vi "main.vi"() -> ()   [LabVIEW 2009]
uses:
  subvi/activity_info.vi
  <vilib>/Utility/file.llb/Write To Spreadsheet File (DBL).vi
  <vilib>/Utility/sysdir.llb/System Directory Type.ctl
panel:
  in  "Do ANN analysis":bool
  in  "Analysis Upperbound (minutes)":dbl(slide)=1000.0 scale=0.0..30.0
  out "minutes left":dbl
  out "minutes of execution":dbl
  out "case 3":i32
  out "case 2":i32
  out "case 1":i32
  out "case 0":i32
  out "output 2":dbl[](array[slide]) scale=0.0..1.0
  out "Correlations":cluster{dbl[], "correlation array":dbl[]}(graph)
  in  "Slide":cluster{dbl, dbl}(slide)={0.0, 1.0} scale=0.0..1.0
  out "above threshold":dbl(slide) scale=0.0..1.0
  in  "Threshold":dbl(slide)=0.85 scale=0.0..1.0
  out "Analyzing":u8(slide) scale=0.0..100.0
  in  "analyze correlations":bool
  in  "Reference Signal":i32
  in  "Reference Signals":dbl[][](array[numeric])
  in  "Save Signal":bool
  in  "read weights":bool
  out "max amplitude":dbl(slide) scale=0.0..4.0
  in  "Path":path=path "E:/Sensor/data/Phase II Data/csv format/Ara/Ara Walking.csv"
  out "C":bool
  out "B":bool
  out "A":bool
  in  "write data":bool
  out "Fundamental frequency":dbl(slide) scale=0.0..6.0
  in  "Normalize":bool
  out "high":bool
  out "med":bool
  out "low":bool
  out "RMS":dbl(slide) scale=0.0..10.0
  in  "write to memory":bool
  out "activity output":u16(ring) items=["A", "B", "C", "D"]
  out "output":dbl[](array[slide]) scale=0.0..1.0
  in  "stop learning":bool
  out "Error (training)":dbl(graph)
  in  "Learning Rate":dbl(slide)=0.336734693877551 scale=0.0..1.0
  in  "Beta":dbl(slide)=1.0 scale=0.0..1.0
  in  "train":bool
  in  "Number of hidden neurons":i32(slide)=9 scale=0.0..20.0
  in  "delete state":bool
  in  "state":u32
  in  "activity":u16(ring) items=["A", "B", "C", "D", "E", "F", "G", "H"]
  in  "save state":bool
  in  "Tab Control":T1(tab)=enum."FFT on data 1"
  out "Time data on X',Y',Z'":T2(graph)
  out "FFT on X',Y',Z'":T3(graph)
  out "Filtered signal":dbl[](graph)
  out "Magnitude of time data":cluster{dbl[], dbl[]}(graph)
  out "activity states":T4(graph)
  in  "Sensor":u16(ring)=1 items=["Sensor 1", "Sensor 2", "Sensor 3"]
  in  "Sensor Type":u16(ring) items=["Acceleration", "Rotation"]
  in  "Sensor Brand":u16(ring)=1 items=["ADXL", "Kinetisense"]
  in  "End time (s) 1":dbl(slide)=10.0 scale=0.0..600.0
  in  "FFT interval (s) 1":dbl(slide)=4.0 scale=0.0..40.0
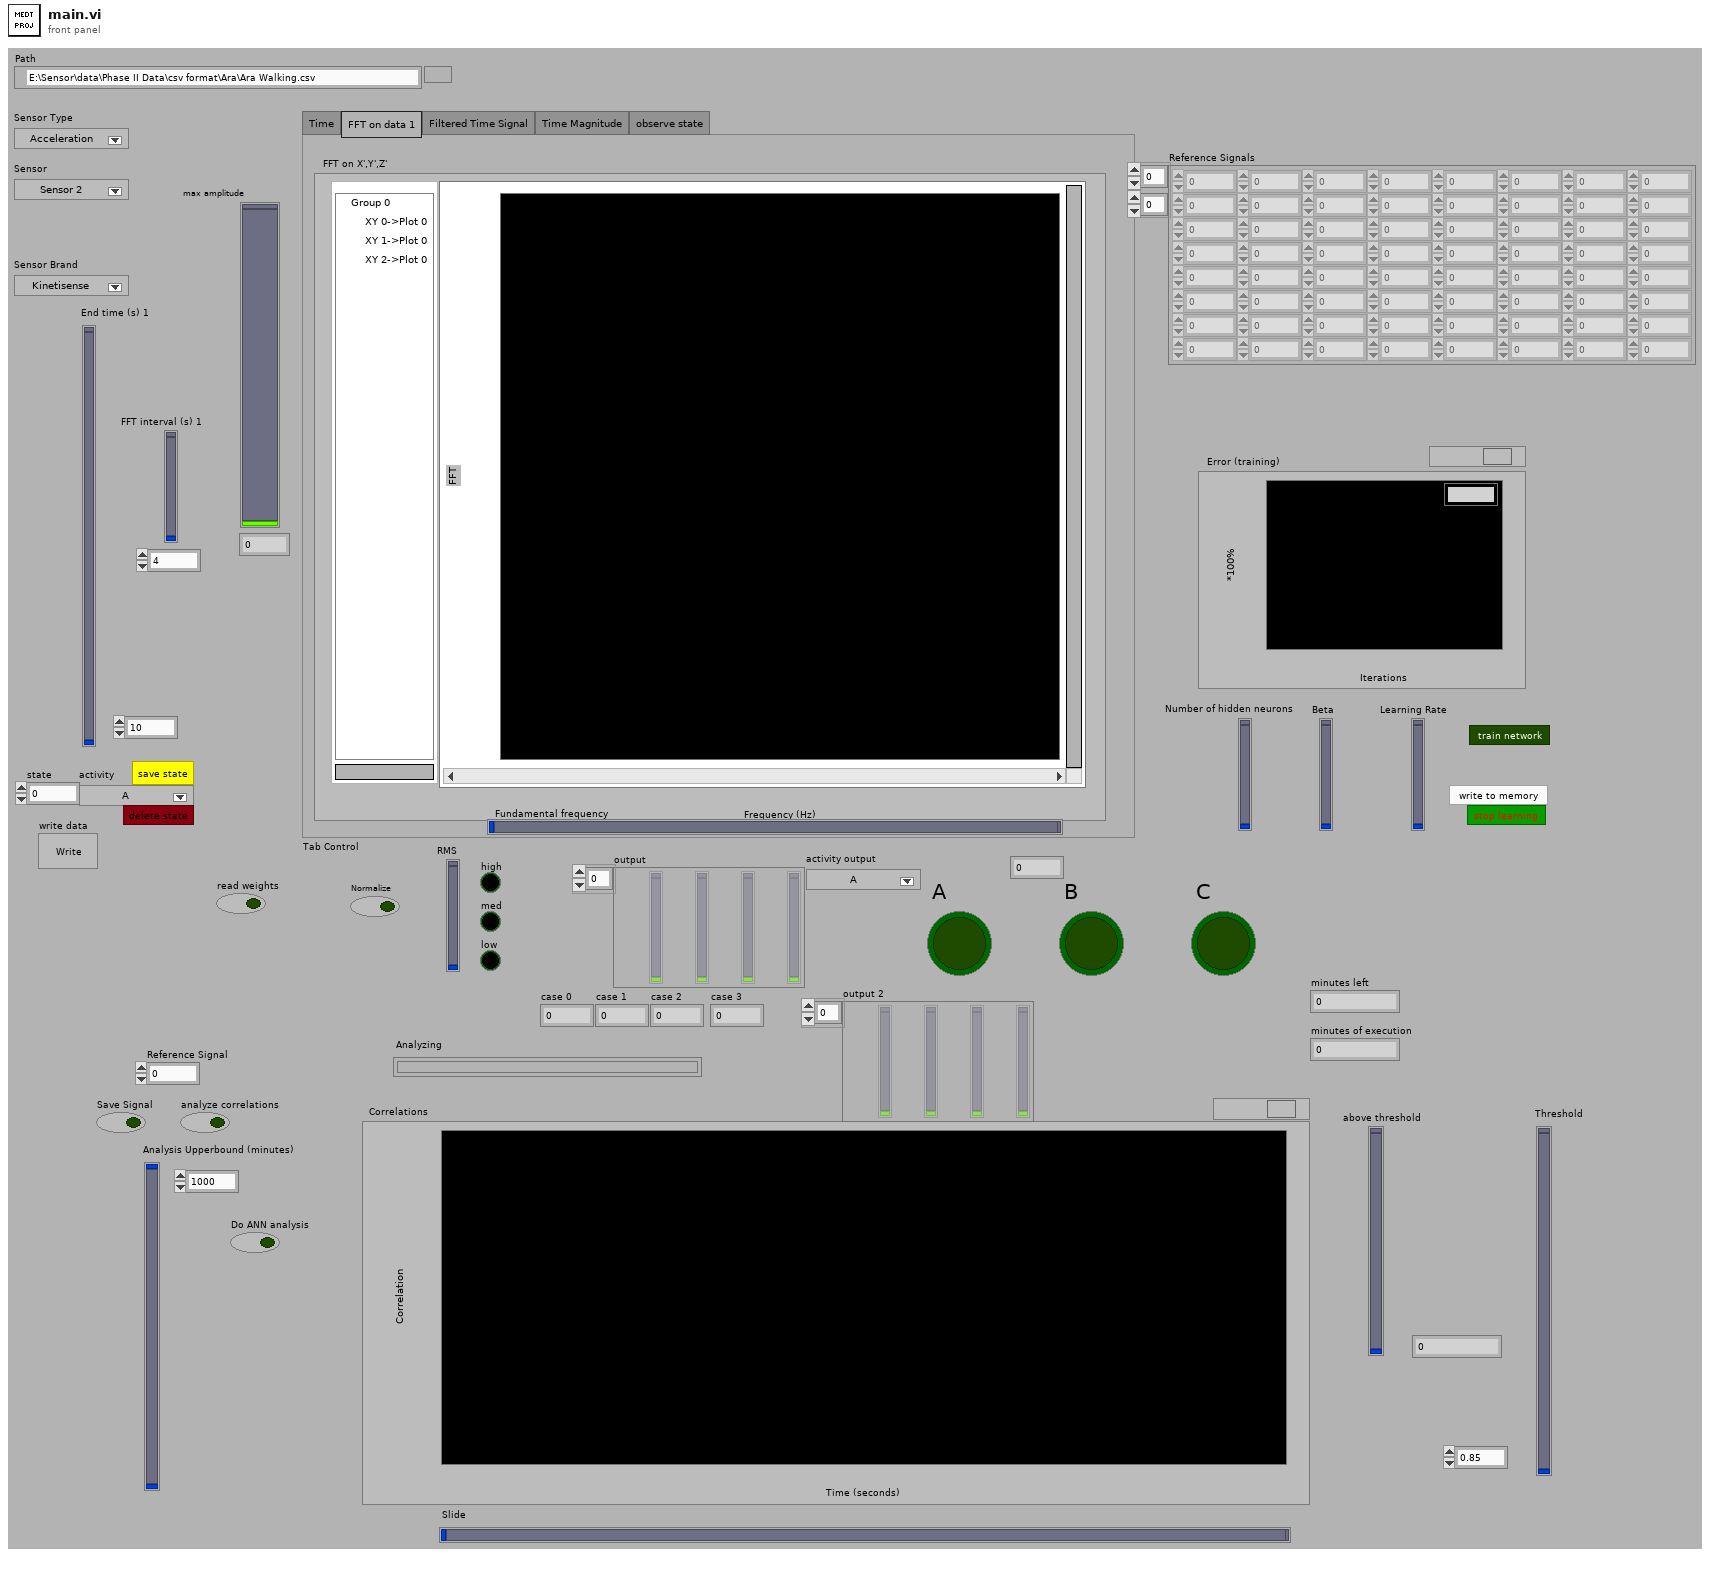
[diagram p1: front panel]
types:
  T1 = enum32{"Time", "FFT on data 1", "Filtered Time Signal", "Time Magnitude", "observe state"}
  T2 = cluster{cluster{dbl[], "Data out":dbl[]}, cluster{dbl[], "Data out":dbl[]}, cluster{dbl[], "Data out":dbl[]}}
  T3 = cluster{"XY Graph":cluster{dbl[], "magnitude":dbl[]}, "XY Graph":cluster{dbl[], "magnitude":dbl[]}, "XY Graph":cluster{dbl[], "magnitude":dbl[]}}
  T4 = cluster{cluster{dbl[], "Bicycling":dbl[]}, cluster{dbl[], "Bicycling":dbl[]}, cluster{dbl[], dbl[]}, cluster{dbl[], dbl[]}, cluster{dbl[], dbl[]}}
  T5 = typedef "System Directory Type.ctl" = i32
  T6 = cluster{"A":dbl[][], "B":dbl[][], "C":dbl[][], "D":dbl[][]}
  T7 = cluster{cluster{dbl[], dbl[]}, cluster{dbl[], dbl[]}, cluster{dbl[], dbl[]}}
  T8 = cluster{"Cluster":cluster{dbl[], "activity":dbl[]}, "Cluster":cluster{dbl[], "activity":dbl[]}, cluster{dbl[], dbl[]}, cluster{dbl[], dbl[]}, cluster{dbl[], dbl[]}}
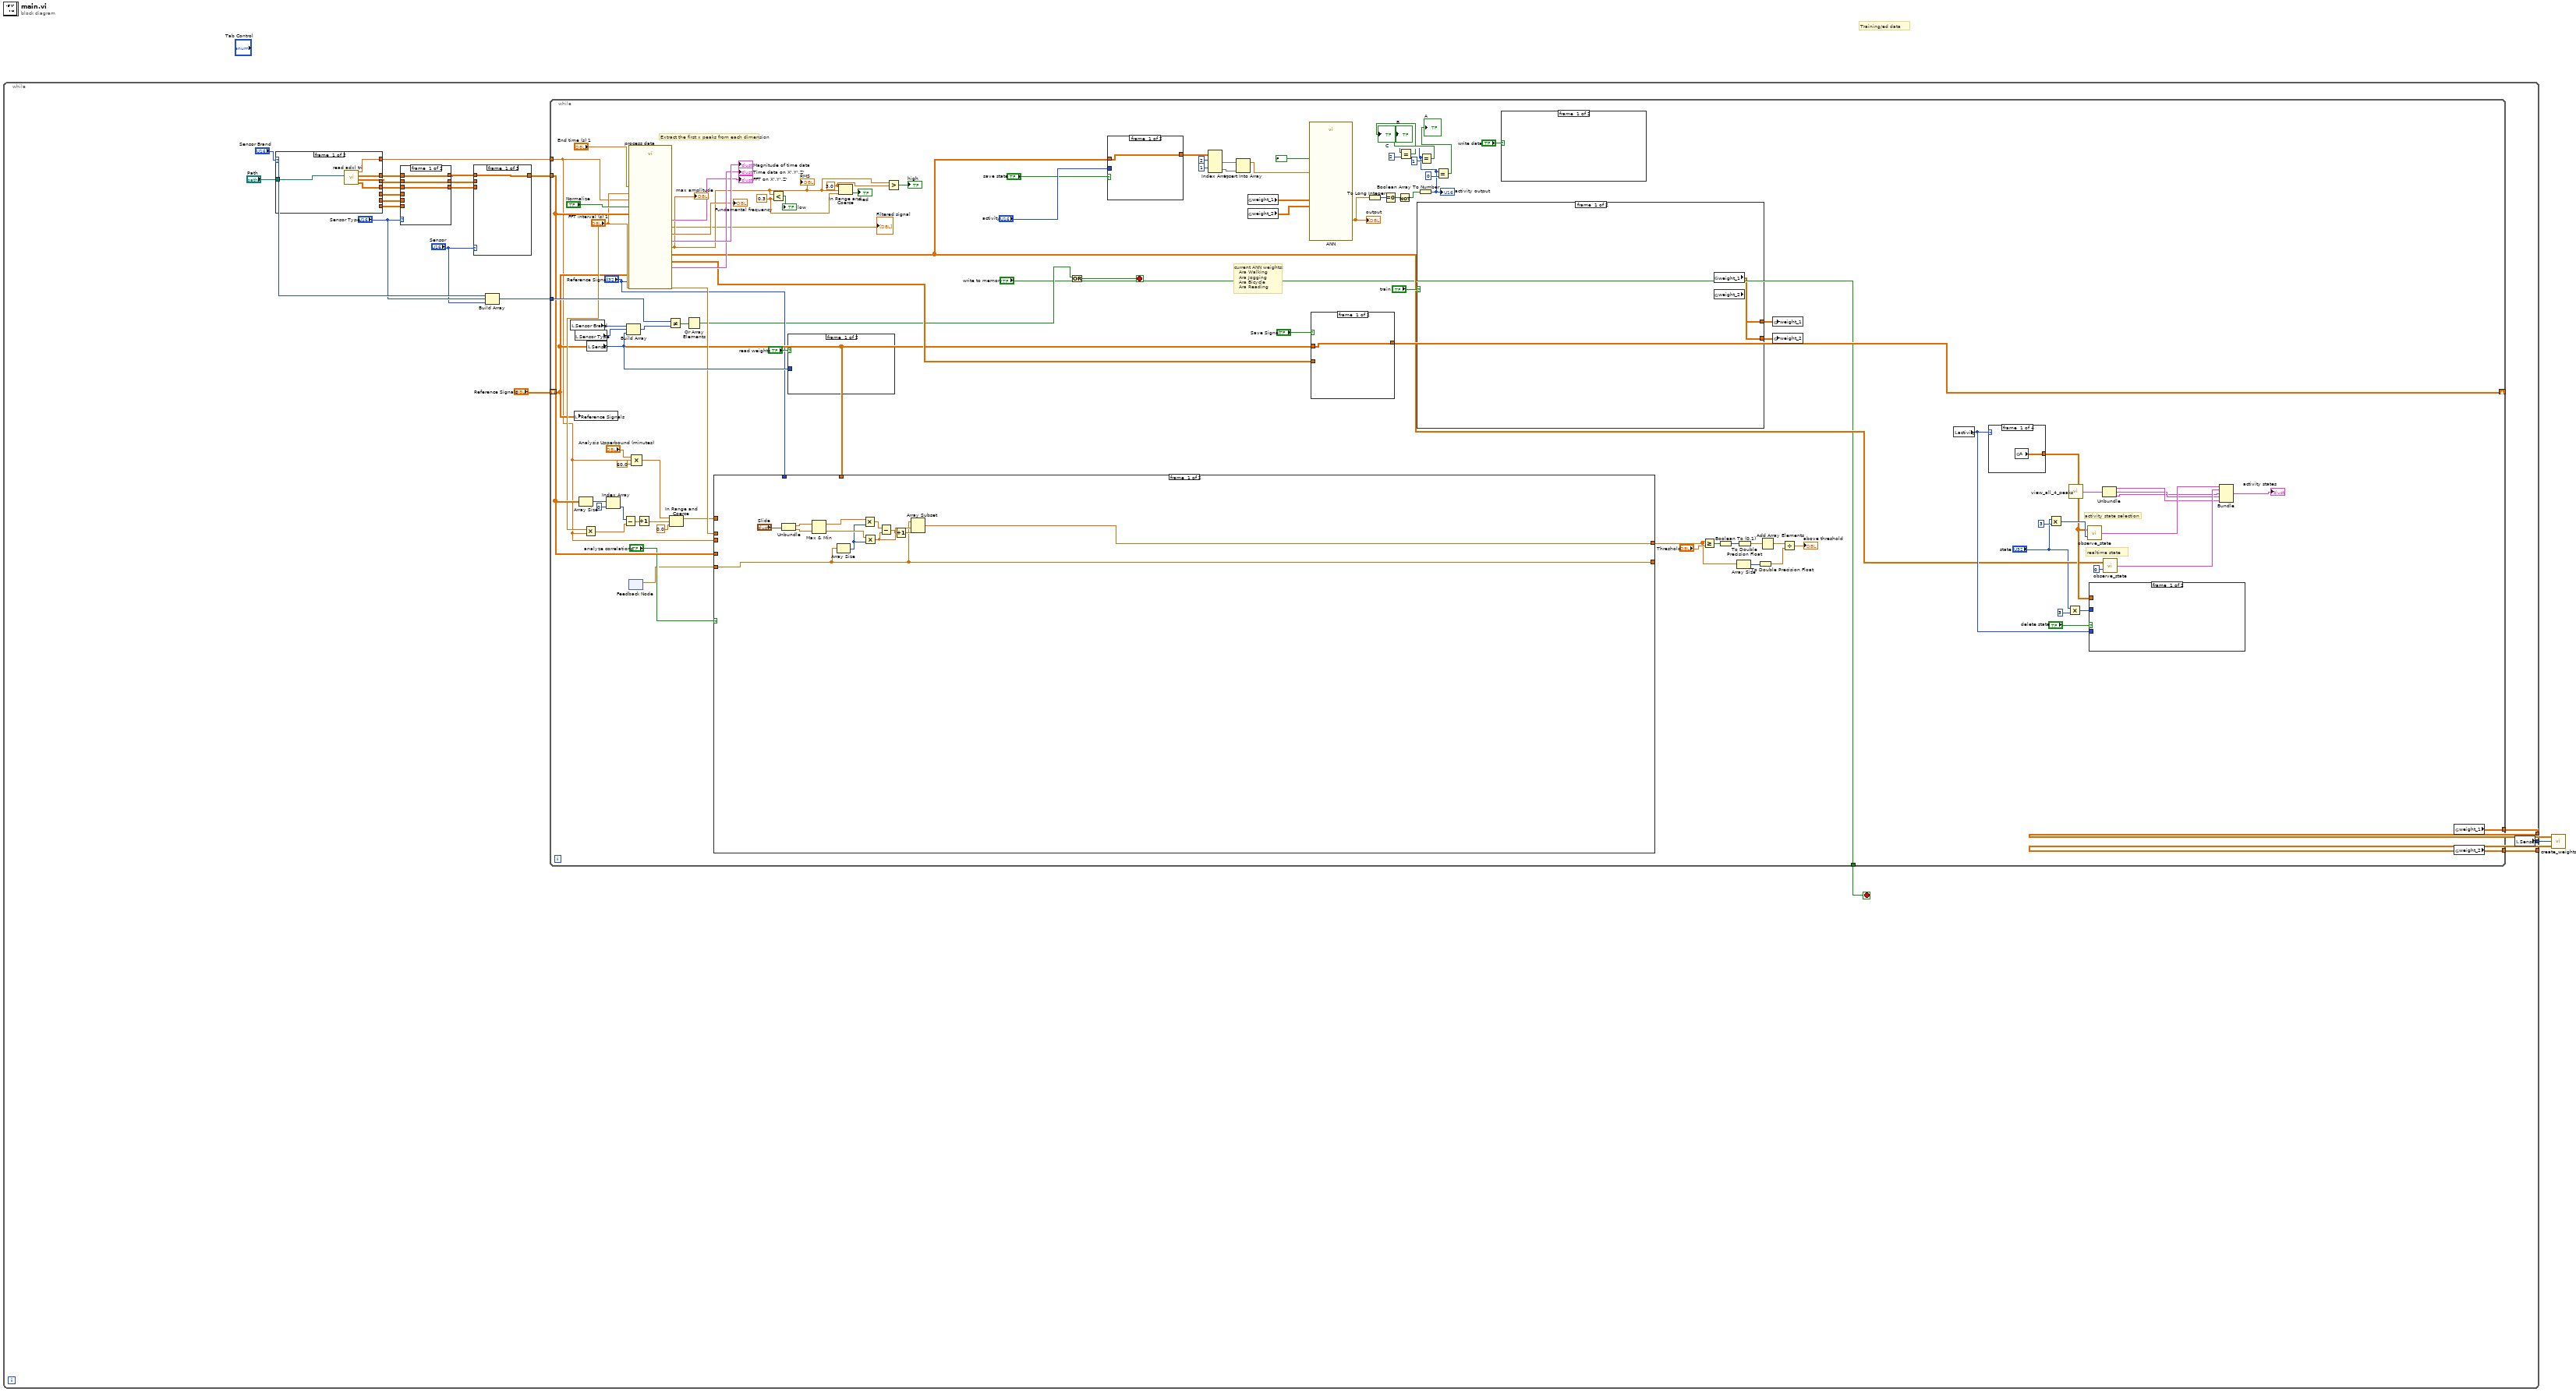
[diagram p0: block diagram]
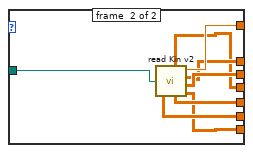
[diagram p5: hidden frame]
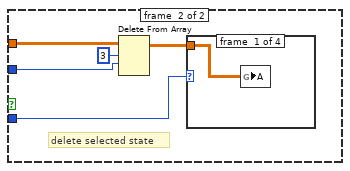
[diagram p6: hidden frame]
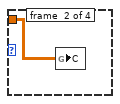
[diagram p7: hidden frame]
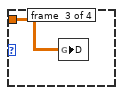
[diagram p8: hidden frame]
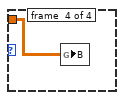
[diagram p9: hidden frame]
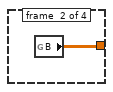
[diagram p10: hidden frame]
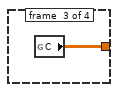
[diagram p11: hidden frame]
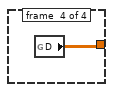
[diagram p12: hidden frame]
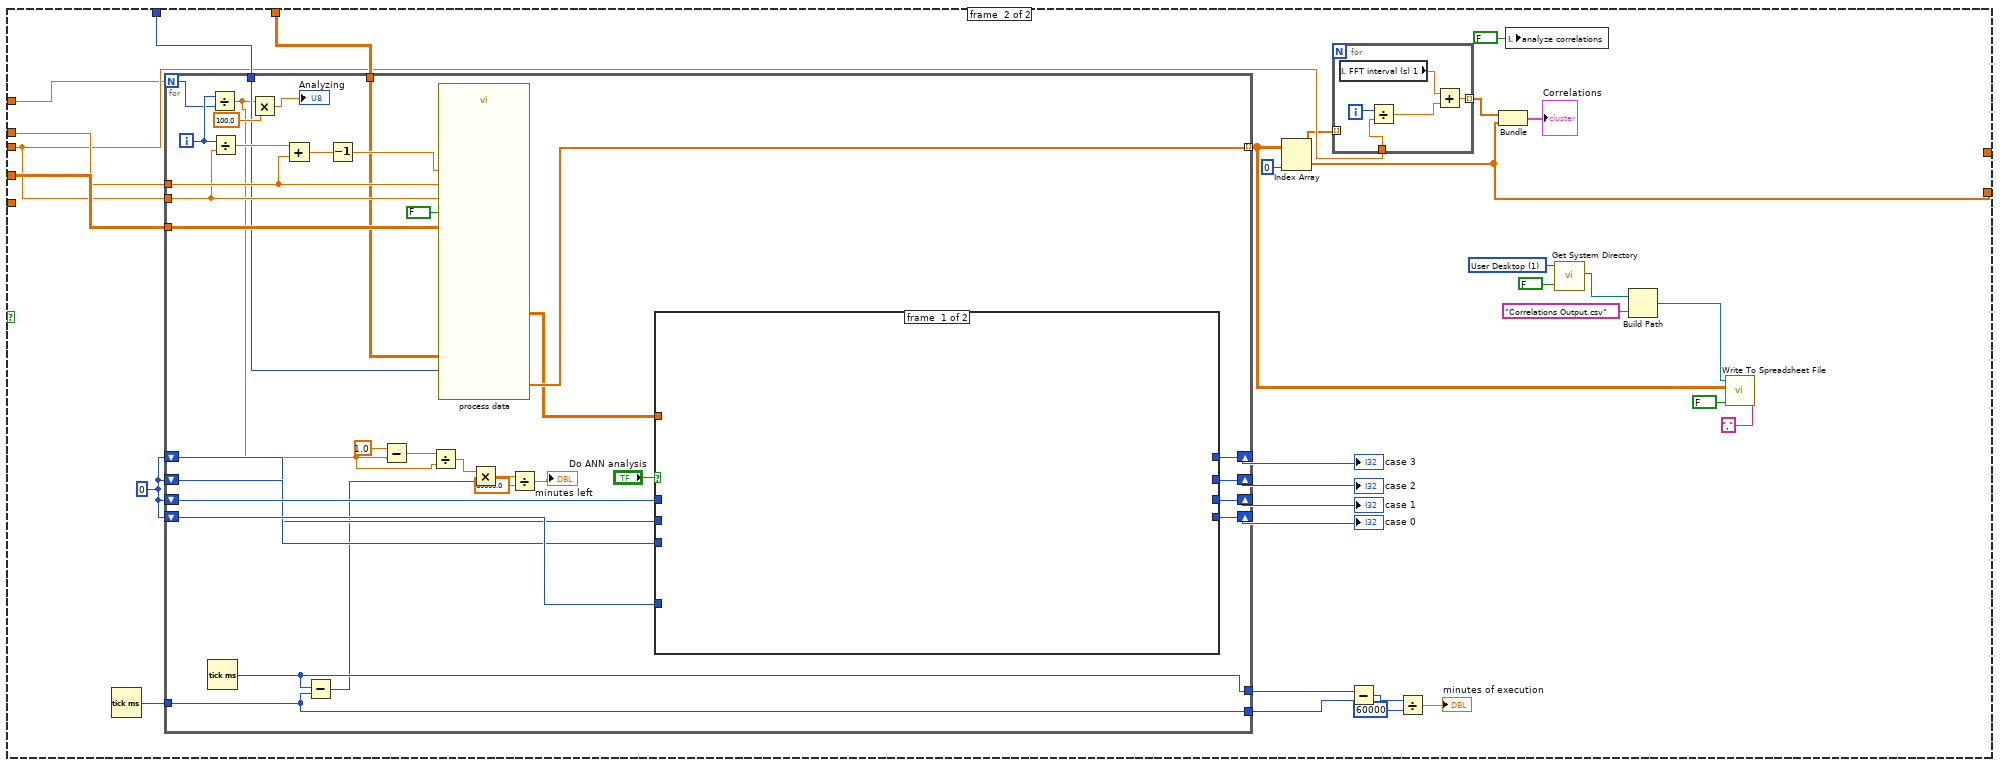
[diagram p13: hidden frame]
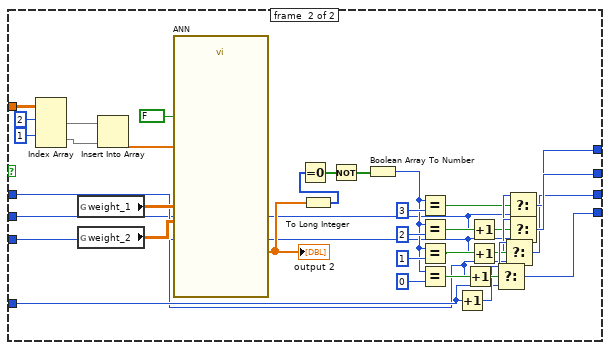
[diagram p14: hidden frame]
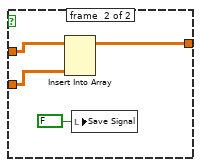
[diagram p15: hidden frame]
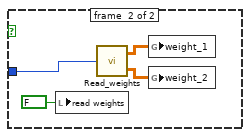
[diagram p16: hidden frame]
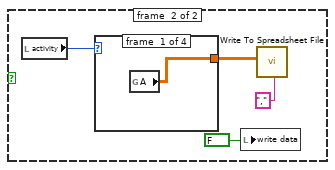
[diagram p17: hidden frame]
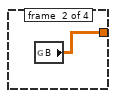
[diagram p18: hidden frame]
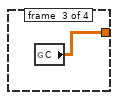
[diagram p19: hidden frame]
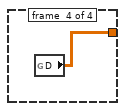
[diagram p20: hidden frame]
diagram:
  # "Training/ed data"
  n1 = while {
    tunnel: [w5] -> w3
    tunnel: [w4] -> w2
    tunnel: [w20] -> w1
    stop <- w21 stop-if-true
    n2 = case shown="1" "Sensor Brand" {
      tunnel: [w38 w46] -> w24
      tunnel: [w37 w45] -> w18
      tunnel: [w36 w44] -> w19
      tunnel: [w35 w43] -> w17
      tunnel: [_ w42] -> w16
      tunnel: [_ w41] -> w15
      tunnel: [_ w40] -> w14
      tunnel: "Path" -> [w34 w39]
      frame #0 {
        n3 = call "read adxl tri.vi"("file path"=w34) -> ("sensor 3 acceleration"=w35:dbl[][], "sensor 2 acceleration"=w37:dbl[][], "sensor 1 acceleration"=w36:dbl[][], "Frequency (Hz)"=w38:dbl)  [unwired: 4 in]
      }
      frame #1 {
        n4 = call "read Kin v2.vi"("file path"=w39) -> ("sensor 3 rotation"=w40:dbl[][], "sensor 1 rotation"=w42:dbl[][], "sensor 2 acceleration"=w45:dbl[][], "sensor 1 acceleration"=w44:dbl[][], "sensor 3 acceleration"=w43:dbl[][], "Frequency (Hz)"=w46:dbl, "sensor 2 rotation"=w41:dbl[][])  [unwired: 1 in]
      }
    }
    n5 = case shown="0, Default" "Sensor Type" {
      tunnel: w19 -> [w30 _]
      tunnel: w18 -> [w29 _]
      tunnel: w17 -> [w28 _]
      tunnel: w16 -> [_ w33]
      tunnel: w15 -> [_ w32]
      tunnel: w14 -> [_ w31]
      tunnel: [w30 w33] -> w8
      tunnel: [w29 w32] -> w13
      tunnel: [w28 w31] -> w12
      frame #0 {
      }
      frame #1 {
      }
    }
    n6 = case shown="1" "Sensor" {
      tunnel: w8 -> [w25 _ _]
      tunnel: w13 -> [_ w26 _]
      tunnel: w12 -> [_ _ w27]
      tunnel: [w25 w26 w27] -> w23
      frame #0 {
      }
      frame #1 {
      }
      frame #2 {
      }
    }
    n7 = Build Array("Sensor Brand", "Sensor Type", "Sensor") -> (w22:u16[])
    n8 = while {
      tunnel: w24 -> [w52]
      tunnel: w23 -> [w95]
      tunnel: w22 -> [w137]
      tunnel: ["write to memory"] -> w21
      shift-right: [w97] -> _
      shift-left: "Reference Signals" -> [w88]
      tunnel: [w56] -> w5
      tunnel: [w55] -> w4
      stop <- w118 stop-if-true
      w114 = 3.0 ("upper limit")
      w116 = 0.3 ("y")
      # "activity state selection"
      # "realtime state"
      # "current ANN weights:\n   Ara Walking\n   Ara Jogging\n   Ara Bicycle\n   Ara Reading"
      # "Extract the first x peaks from each dimension"
      n9 = local read "Sensor Brand"() -> (w141:u16)
      n10 = local write "Reference Signals"(w88) -> ()
      n11 = local read "Sensor Type"() -> (w140:u16)
      n12 = Array Size(array=w95) -> (size(s)=w94:i32[])
      n13 = Multiply(x="FFT interval (s) 1", y=w52) -> (x*y=w91:dbl)
      n14 = local read "Sensor"() -> (w100:u16)
      n15 = Index Array(array=w94, index=0) -> (element=w90:i32)
      n16 = Subtract(x=w90, y=w91) -> (x-y=w89:dbl)
      n17 = Build Array(w141, w140, w100) -> (w139:u16[])
      n18 = call "process data.vi"("Frequency (Hz)"=w52, "Reference Signal"="Reference Signal", "sensor input"=w95, "In Signals"=w88, "FFT interval (s)"="FFT interval (s) 1", "Normalize"="Normalize", "End time (s)"="End time (s) 1") -> ("Fundamental frequency"=→"Fundamental frequency":dbl, "FFT"=→"FFT on X',Y',Z'":T3, "peaks"=w60:dbl[][], "Magnitude of time data"=→"Magnitude of time data":cluster{dbl[], dbl[]}, "x',y',z'"=→"Time data on X',Y',Z'":T2, "Signals"=w96:dbl[][], "Filtered signal"=→"Filtered signal":dbl[], "max amplitude"=w102:dbl)  [unwired: 1 out]
      "RMS" <- w102
      "max amplitude" <- w102
      n19 = feedback #1() -> (w76:dbl[])  [unwired: 1 in]
      n20 = Compound Arithmetic op=MULTIPLY("Analysis Upperbound (minutes)", w52, 60.0 ("value")) -> (w48:dbl)
      n21 = Increment(x=w89) -> (x+1=w50:dbl)
      n22 = Not Equal?(x=w137, y=w139) -> (x != y?=w138:bool[])
      n23 = In Range and Coerce(upper limit=w48, x=w50, lower limit=0.0) -> (coerced(x)=w47:dbl)  [unwired: 1 out]
      n24 = Or Array Elements(Boolean array=w138) -> (logical OR=w61:bool)
      n25 = case shown="True" "analyze correlations" {
        tunnel: w95 -> [_ w200]
        tunnel: w52 -> [_ w194]
        tunnel: "FFT interval (s) 1" -> [_ w199]
        tunnel: w47 -> [_ w190]
        tunnel: w88 -> [_ w198]
        tunnel: "Reference Signal" -> [_ w195]
        tunnel: [w160 w193] -> w77
        tunnel: w76 -> [w160 _]
        tunnel: [w159 _] -> w75
        frame #0 {
          n26 = Unbundle("Slide") -> (w169:dbl, w168:dbl)
          n27 = Max & Min(x=w169, y=w168) -> (max(x,y)=w165:dbl, min(x,y)=w167:dbl)
          n28 = Array Size(array=w160) -> (size(s)=w166:i32)
          n29 = Multiply(x=w165, y=w166) -> (x*y=w164:dbl)
          n30 = Multiply(x=w167, y=w166) -> (x*y=w163:dbl)
          n31 = Subtract(x=w164, y=w163) -> (x-y=w161:dbl)
          n32 = Increment(x=w161) -> (x+1=w162:dbl)
          n33 = Array Subset(array=w160, index=w163, length=w162) -> (w159:dbl[])
        }
        frame #1 {
          w175 = T5 1 items=["User Home", "User Desktop", "User Documents", "User Application Data", "User Preferences", "User Temporary", "Public Documents", "Public Application Data", "Public Preferences", "System Core Libraries", "System Installed Libraries", "Application Files", "Boot Volume Root"] ("system directory type")
          w189 = 0
          n34 = Tick Count (ms)() -> (millisecond timer value=w184:u32)
          n35 = for {
            N: w190 -> [w229]
            tunnel: w200 -> [w238]
            tunnel: w199 -> [w236]
            tunnel: w194 -> [w235]
            tunnel: [w237] -> w178 mode=indexing
            tunnel: w198 -> [w231]
            tunnel: w195 -> [w226]
            shift-right: [w223] -> w188
            shift-left: w189 -> [w224]
            shift-right: [w217] -> w187
            shift-left: w189 -> [w222]
            shift-right: [w220] -> w186
            shift-left: w189 -> [w221]
            shift-right: [w218] -> w185
            shift-left: w189 -> [w219]
            tunnel: w184 -> [w215]
            tunnel: [w215] -> w183
            tunnel: [w216] -> w179
            i -> [w230]
            n36 = Tick Count (ms)() -> (millisecond timer value=w216:u32)
            n37 = Divide(x=w230, y=w229) -> (x/y=w212:dbl)
            n38 = Divide(x=w230, y=w235) -> (x/y=w234:dbl)
            n39 = Multiply(x=w212, y=100.0) -> (x*y=→"Analyzing":dbl)
            n40 = Add(x=w234, y=w236) -> (x+y=w233:dbl)
            n41 = Subtract(x=w216, y=w215) -> (x-y=w210:u32)
            n42 = Decrement(x=w233) -> (x-1=w232:dbl)
            n43 = Subtract(x=1.0, y=w212) -> (x-y=w213:dbl)
            n44 = Divide(x=w213, y=w212) -> (x/y=w211:dbl)
            n45 = call "process data.vi"("Frequency (Hz)"=w235, "Reference Signal"=w226, "sensor input"=w238, "In Signals"=w231, "FFT interval (s)"=w236, "Normalize"=FALSE, "End time (s)"=w232) -> ("peaks"=w225:dbl[][], "correlation array"=w237:dbl[])  [unwired: 7 out]
            n46 = Multiply(x=w211, y=w210) -> (x*y=w209:dbl)
            n47 = Divide(x=w209, y=60000.0) -> (x/y=→"minutes left":dbl)
            n48 = case shown="True" "Do ANN analysis" {
              tunnel: w225 -> [_ w264]
              tunnel: w224 -> [_ w253]
              tunnel: [_ w252] -> w223
              tunnel: w222 -> [_ w249]
              tunnel: w221 -> [_ w246]
              tunnel: [_ w245] -> w220
              tunnel: w219 -> [_ w242]
              tunnel: [_ w241] -> w218
              tunnel: [_ w240] -> w217
              frame #0 {
              }
              frame #1 {
                n49 = Index Array(array=w264, index (row) #1=2 ("index (row)"), index (row) #2=1 ("index (row)")) -> (element #1=w270:dbl[], element #2=w269:dbl[])  [unwired: 2 in]
                n50 = global read "activity_info.vi" "weight_1"() -> (w267:dbl[][])
                n51 = global read "activity_info.vi" "weight_2"() -> (w266:dbl[][])
                n52 = Insert Into Array(array=w270, new element=w269) -> (w268:dbl[])  [unwired: 1 in]
                n53 = call "ANN.vi"("Input"=w268, "Weight_2"=w266, "Weight_1"=w267, "Back Propagation"=FALSE) -> ("output"=w265:dbl[])  [unwired: 8 in, 3 out]
                "output 2" <- w265
                n54 = To Long Integer(number=w265) -> (32bit integer=w262:i32[])
                n55 = Equal To 0?(x=w262) -> (x = 0?=w263:bool[])
                n56 = Not(x=w263) -> (.not. x?=w261:bool[])
                n57 = Boolean Array To Number(Boolean array=w261) -> (number=w256:u32)
                n58 = Equal?(x=w256, y=3) -> (x = y?=w243:bool)
                n59 = Equal?(x=w256, y=2) -> (x = y?=w247:bool)
                n60 = Equal?(x=w256, y=1) -> (x = y?=w250:bool)
                n61 = Equal?(x=w256, y=0) -> (x = y?=w255:bool)
                n62 = Increment(x=w253) -> (x+1=w254:i32)
                n63 = Increment(x=w249) -> (x+1=w251:i32)
                n64 = Increment(x=w242) -> (x+1=w244:i32)
                n65 = Increment(x=w246) -> (x+1=w248:i32)
                n66 = Select(t=w254, s=w255, f=w253) -> (s? t:f=w252:i32)
                n67 = Select(t=w251, s=w250, f=w249) -> (s? t:f=w240:i32)
                n68 = Select(t=w244, s=w243, f=w242) -> (s? t:f=w241:i32)
                n69 = Select(t=w248, s=w247, f=w246) -> (s? t:f=w245:i32)
              }
            }
          }
          "case 0" <- w188
          "case 1" <- w187
          "case 2" <- w186
          "case 3" <- w185
          n70 = Index Array(array=w178, index (col)=0 ("disabled index (col)")) -> (element=w193:dbl[])  [unwired: 1 in]
          n71 = for {
            tunnel: w193 -> [_] mode=indexing
            tunnel: w194 -> [w204]
            tunnel: [w201] -> w191 mode=indexing
            i -> [w205]
            n72 = local read "FFT interval (s) 1"() -> (w202:dbl)
            n73 = Divide(x=w205, y=w204) -> (x/y=w203:dbl)
            n74 = Add(x=w202, y=w203) -> (x+y=w201:dbl)
          }
          n75 = Subtract(x=w179, y=w183) -> (x-y=w182:u32)
          n76 = Divide(x=w182, y=u32 60000) -> (x/y=→"minutes of execution":dbl)
          n77 = Bundle(w191, "correlation array"=w193) -> (→"Correlations":cluster{dbl[], "correlation array":dbl[]})  [unwired: 1 in]
          n78 = local write "analyze correlations"(FALSE ("analyze correlations")) -> ()
          n79 = call <vilib>:"Get System Directory.vi"("create directory if not found? (F)"=FALSE, "system directory type"=w175) -> ("system directory"=w173:path)  [unwired: 9 in]
          n80 = Build Path(base path=w173, name or relative path="Correlations Output.csv") -> (appended path=w172:path)
          n81 = call-poly <vilib>:"Write To Spreadsheet File.vi"("delimiter (\\t)"="," ("delimiter (\\t)"), "append to file? (new file:F)"=FALSE, "2D data"=w178, "file path (dialog if empty)"=w172) -> ()  [unwired: 4 in, 1 out]
        }
      }
      n82 = Less?(x=w102, y=w116) -> (x < y?=→"low":bool)
      n83 = case shown="True" "read weights" {
        tunnel: w100 -> [_ w282]
        frame #0 {
        }
        frame #1 {
          n84 = local write "read weights"(FALSE ("read weights")) -> ()
          n85 = call "Read_weights.vi"("sensor"=w282) -> ("weights 1"=w280:dbl[][], "weights 2"=w279:dbl[][])
          n86 = global write "activity_info.vi" "weight_1"(w280) -> ()
          n87 = global write "activity_info.vi" "weight_2"(w279) -> ()
        }
      }
      n88 = In Range and Coerce(upper limit=w114, x=w102, lower limit=w116) -> (In Range?=→"med":bool)  [unwired: 1 out]
      n89 = Greater?(x=w102, y=w114) -> (0:→"high":bool)
      n90 = Or(x=w61, y="write to memory") -> (x .or. y?=w118:bool)
      n91 = case shown="True" "save state" {
        tunnel: w60 -> [w314 w316]
        tunnel: [w314 w316] -> w128
        tunnel: "activity" -> [_ w315]
        frame #0 {
        }
        frame #1 {
          # "save the state to  temp memory"
          n92 = call "save_state.vi"("state"=w315, "peaks"=w316) -> ()  [unwired: 1 in]
        }
      }
      n93 = Index Array(array=w128, index (row) #1=2 ("index (row)"), index (row) #2=1 ("index (row)")) -> (element #1=w131:dbl[], element #2=w130:dbl[])  [unwired: 2 in]
      n94 = Insert Into Array(array=w131, new element=w130) -> (w129:dbl[])  [unwired: 1 in]
      n95 = global read "activity_info.vi" "weight_1"() -> (w127:dbl[][])
      n96 = global read "activity_info.vi" "weight_2"() -> (w126:dbl[][])
      n97 = call "ANN.vi"("Input"=w129, "Weight_2"=w126, "Weight_1"=w127, "Back Propagation"=FALSE) -> ("output"=w122:dbl[])  [unwired: 8 in, 3 out]
      "output" <- w122
      n98 = case shown="True" "Save Signal" {
        tunnel: w96 -> [_ w278]
        tunnel: [w274 w275] -> w97
        tunnel: w88 -> [w274 w276]
        frame #0 {
        }
        frame #1 {
          n99 = Insert Into Array(array=w276, new element=w278) -> (w275:dbl[][])  [unwired: 2 in]
          n100 = local write "Save Signal"(FALSE ("Save Signal")) -> ()
        }
      }
      n101 = To Long Integer(number=w122) -> (32bit integer=w121:i32[])
      n102 = Equal To 0?(x=w121) -> (x = 0?=w120:bool[])
      n103 = Not(x=w120) -> (.not. x?=w119:bool[])
      n104 = case shown="True" "train" {
        tunnel: [w291 w296] -> w125
        tunnel: [w292 w295] -> w124
        frame #0 {
          n105 = global read "activity_info.vi" "weight_1"() -> (w292:dbl[][])
          n106 = global read "activity_info.vi" "weight_2"() -> (w291:dbl[][])
        }
        frame #1 {
          # "# of inputs +1"
          # "# of outputs"
          n107 = call "initial weights.vi"("Number of classifiers"=3, "Number of hidden neurons"="Number of hidden neurons", "Inputs + 1"=9) -> ("Weights 2"=w304:dbl[][], "Weights 1"=w303:dbl[][])
          n108 = global read "activity_info.vi" "D"() -> (w297:dbl[][])
          n109 = global read "activity_info.vi" "C"() -> (w301:dbl[][])
          n110 = global read "activity_info.vi" "B"() -> (w300:dbl[][])
          n111 = global read "activity_info.vi" "A"() -> (w294:dbl[][])
          n112 = Bundle("A"=w294, "B"=w300, "C"=w301, "D"=w297) -> (w302:T6)  [unwired: 1 in]
          n113 = while {
            tunnel: w302 -> [w305]
            shift-right: [w311] -> w295
            shift-left: w303 -> [w313]
            shift-right: [w310] -> w296
            shift-left: w304 -> [w312]
            stop <- "stop learning" stop-if-true
            n114 = call "learning_phase.vi"("Weights 2"=w312, "Weights 1"=w313, "Learning Rate"="Learning Rate", "Beta"="Beta", "inputs"=w305) -> ("Error"=→"Error (training)":dbl, "Weight_2_out"=w310:dbl[][], "Weight_1_out"=w311:dbl[][])
          }
        }
      }
      n115 = Boolean Array To Number(Boolean array=w119) -> (number=w105:u32)
      "activity output" <- w105
      n116 = Equal?(x=w105, y=u32 2) -> (x = y?=→"C":bool)
      n117 = Equal?(x=w105, y=u32 1) -> (x = y?=→"B":bool)
      n118 = Equal?(x=w105, y=u32 0) -> (x = y?=→"A":bool)
      n119 = case shown="True" "write data" {
        frame #0 {
        }
        frame #1 {
          n120 = local read "activity"() -> (w286:u16)
          n121 = case shown="0, Default" w286 {
            tunnel: [w287 w288 w289 w290] -> w285
            frame #0 {
              n122 = global read "activity_info.vi" "A"() -> (w287:dbl[][])
            }
            frame #1 {
              n123 = global read "activity_info.vi" "B"() -> (w288:dbl[][])
            }
            frame #2 {
              n124 = global read "activity_info.vi" "C"() -> (w289:dbl[][])
            }
            frame #3 {
              n125 = global read "activity_info.vi" "D"() -> (w290:dbl[][])
            }
          }
          n126 = local write "write data"(FALSE ("write data")) -> ()
          n127 = call-poly <vilib>:"Write To Spreadsheet File.vi"("delimiter (\\t)"="," ("delimiter (\\t)"), "2D data"=w285) -> ()  [unwired: 6 in, 1 out]
        }
      }
      n128 = Greater Or Equal?(x=w75, y="Threshold") -> (x >= y?=w79:bool[])
      n129 = Boolean To (0,1)(Boolean=w79) -> (0, 1=w80:i16[])
      n130 = Array Size(array=w75) -> (size(s)=w83:i32)
      n131 = To Double Precision Float(number=w80) -> (double precision float=w81:dbl[])
      n132 = To Double Precision Float(number=w83) -> (double precision float=w84:dbl)
      n133 = Add Array Elements(numeric array=w81) -> (sum=w82:dbl)
      n134 = global write "activity_info.vi" "weight_1"(w124) -> ()
      n135 = global write "activity_info.vi" "weight_2"(w125) -> ()
      n136 = Divide(x=w82, y=w84) -> (x/y=→"above threshold":dbl)
      n137 = local read "activity"() -> (w62:u16)
      n138 = case shown="3" w62 {
        tunnel: [w155 w156 w157 w158] -> w63
        frame #0 {
          n139 = global read "activity_info.vi" "A"() -> (w155:dbl[][])
        }
        frame #1 {
          n140 = global read "activity_info.vi" "B"() -> (w156:dbl[][])
        }
        frame #2 {
          n141 = global read "activity_info.vi" "C"() -> (w157:dbl[][])
        }
        frame #3 {
          n142 = global read "activity_info.vi" "D"() -> (w158:dbl[][])
        }
      }
      n143 = Multiply(x="state", y=u32 3) -> (x*y=w73:u32)
      n144 = Multiply(x="state", y=u32 3) -> (x*y=w70:u32)
      n145 = call "view_all_4_peaks.vi"("activity"=w63) -> ("Cluster"=w67:T7)
      n146 = call "observe_state.vi"("Numeric"=w73, "activity"=w63) -> ("Cluster"=w72:cluster{dbl[], "activity":dbl[]})
      n147 = case shown="True" "delete state" {
        tunnel: w63 -> [_ w150]
        tunnel: w70 -> [_ w148]
        tunnel: w62 -> [_ w147]
        frame #0 {
        }
        frame #1 {
          # "delete selected state"
          n148 = Delete From Array(array=w150, length=3, index (row)=w148) -> (array with subset deleted=w146:dbl[][])  [unwired: 1 in, 1 out]
          n149 = case shown="3" w147 {
            tunnel: w146 -> [w151 w152 w153 w154]
            frame #0 {
              n150 = global write "activity_info.vi" "A"(w151) -> ()
            }
            frame #1 {
              n151 = global write "activity_info.vi" "C"(w152) -> ()
            }
            frame #2 {
              n152 = global write "activity_info.vi" "D"(w153) -> ()
            }
            frame #3 {
              n153 = global write "activity_info.vi" "B"(w154) -> ()
            }
          }
        }
      }
      n154 = Unbundle(w67) -> (w66:cluster{dbl[], dbl[]}, w65:cluster{dbl[], dbl[]}, w64:cluster{dbl[], dbl[]})
      n155 = call "observe_state.vi"("Numeric"=u32 0, "activity"=w60) -> ("Cluster"=w68:cluster{dbl[], "activity":dbl[]})
      n156 = Bundle("Cluster"=w72, "Cluster"=w68, w64, w65, w66) -> (→"activity states":T8)  [unwired: 1 in]
      n157 = global read "activity_info.vi" "weight_1"() -> (w56:dbl[][])
      n158 = global read "activity_info.vi" "weight_2"() -> (w55:dbl[][])
    }
    n159 = local read "Sensor"() -> (w20:u16)
  }
  n160 = call "create_weights.vi"("weight2"=w2, "Ring"=w1, "weight1"=w3) -> ()
